vi "PH_Sixpack_Switch.evt set Remote Controlled.vi"(0 "i ref in":refnum<vi>, 2 "Instance":string="N/A", 3 "Remote Controlled":bool, 5 "error in (no error)":errorcluster) -> (14 "i ref out":refnum<vi>, 19 "error out":errorcluster)   [LabVIEW 2014, in "PH_Sixpack_Switch.lvlib"]
doc: "This VI sends a \"Remote Controlled Command\" in command"
uses:
  PH_Sixpack_Switch.lvlib
  CSCore/CSSystem/CoreLib/CoreLib.short 2 byte array.vi
  CSCore/CSSystem/CoreLib/CoreLib.lvlib
  CSCore/BaseProcess/BaseProcess.lvlib
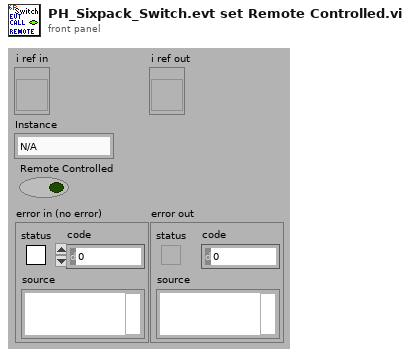
[diagram p1: front panel]
types:
  T1 = typedef "CoreDefs.rawDataType.ctl" = i8[]
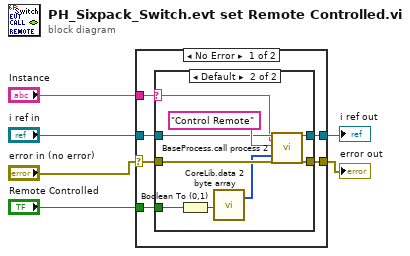
[diagram p0: block diagram]
diagram:
  n1 = case shown="No Error" "error in (no error)" {
    selector: "error in (no error)" -> [w7 w24]
    tunnel: [w12 w25] -> w6
    tunnel: [w11 w24] -> w5
    tunnel: "i ref in" -> [w10 w25]
    tunnel: "Remote Controlled" -> [w9 _]
    tunnel: "Instance" -> [w8 _]
    frame No Error {
      n2 = case shown="Default" w8 {
        selector: w8 -> [_ w15]
        tunnel: [w14 w18] -> w12
        tunnel: [w13 w17] -> w11
        tunnel: w10 -> [w14 w16]
        tunnel: w7 -> [w13 w23]
        tunnel: w9 -> [_ w21]
        frame "N/A" {
        }
        frame Default {
          n3 = Boolean To (0,1)(Boolean=w21) -> (0, 1=w22:i16)
          n4 = call-poly "CoreLib.data 2 byte array.vi"("i16"=w22) -> ("byteArray out"=w20:T1)  [unwired: 18 in]
          n5 = call "BaseProcess.call process 2.vi"("i ref in"=w16, "Object"=w15, "Selector"="Control Remote", "Data"=w20, "error in (no error)"=w23) -> ("i ref out"=w18:refnum<vi>, "error out"=w17:errorcluster)  [unwired: 13 in]
        }
      }
    }
    frame Error {
    }
  }
  "error out" <- w5
  "i ref out" <- w6
